vi "Device Parameters to Configuration Elements.vi"(11 "device parameters":T3) -> (0 "biu number":i32, 1 "card or slot number":i32, 2 "card or slot number caption":string, 3 "initialization method":T4, 4 "bus selection":T2, 6 "coupling mode":T1)   [LabVIEW 2020, in "AIM MIL-STD-1553 System Explorer.lvlib" / "Implementation.lvlib"]
uses:
  Implementation.lvlib
  Scripting/Constants.vi
  Scripting/AIM MIL-STD-1553 Scripting.lvlib
  Shared/Initialization Method.ctl
  Shared/AIM Hardware Parameters.ctl
  Shared/Bus Selection.ctl
  Shared/Coupling Mode.ctl
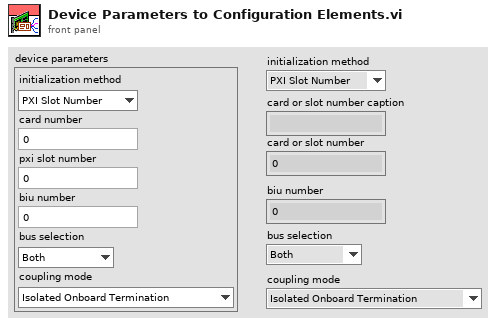
[diagram p1: front panel]
types:
  T1 = typedef "Coupling Mode.ctl" = enum16{"Isolated Onboard Termination", "Transformer Coupled", "Direct Coupled", "External with Onboard Termination", "Onboard Digital Wrap-around"}
  T2 = typedef "Bus Selection.ctl" = enum16{"Both", "Primary", "Secondary"}
  T3 = typedef "AIM Hardware Parameters.ctl" = cluster{"initialization method":T4, "card number":i32, "pxi slot number":i32, "biu number":i32, "bus selection":T2, "coupling mode":T1}
  T4 = typedef "Initialization Method.ctl" = enum16{"PXI Slot Number", "Card Number"}
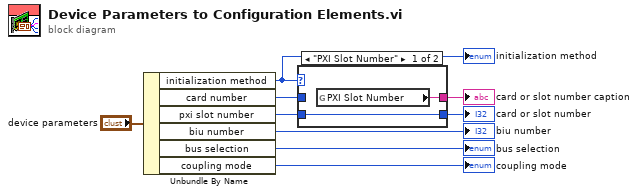
[diagram p0: block diagram]
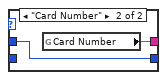
[diagram p2: hidden frame]
diagram:
  n1 = Unbundle By Name("device parameters") -> ("initialization method"=w9:T4, "card number"=w5:i32, "pxi slot number"=w6:i32, "biu number"=→"biu number":i32, "bus selection"=→"bus selection":T2, "coupling mode"=→"coupling mode":T1)
  "initialization method" <- w9
  n2 = case shown="\"PXI Slot Number\"" w9 {
    tunnel: w5 -> [_ w13]
    tunnel: w6 -> [w10 _]
    tunnel: [w10 w13] -> w7
    tunnel: [w11 w12] -> w8
    frame "PXI Slot Number" {
      n3 = global read "Constants.vi" "PXI Slot Number"() -> (w11:string)
    }
    frame "Card Number" {
      n4 = global read "Constants.vi" "Card Number"() -> (w12:string)
    }
  }
  "card or slot number caption" <- w8
  "card or slot number" <- w7
